vi "Init Edge Detector.vi"(6 "Unsee last word":bool=TRUE, 8 "error in (no error)":errorcluster, 11 "Spectrum Recorder too in":refnum<class "Spectrum Recorder too.lvclass">) -> (0 "error out":errorcluster, 3 "Spectrum Recorder too out":refnum<class "Spectrum Recorder too.lvclass">)   [LabVIEW 2018, in "Spectrum Recorder too.lvclass"]
uses:
  Spectrum Recorder too.lvclass
  Spectrum Recorder too.lvclass/Spectrum Recorder too.ctl
  Read RP transceiver.vi
  Write RP transceiver.vi
  NHMFL_Core/Libraries/Red Pitaya/RP Core/RP Transceiver/RP Transceiver.lvclass
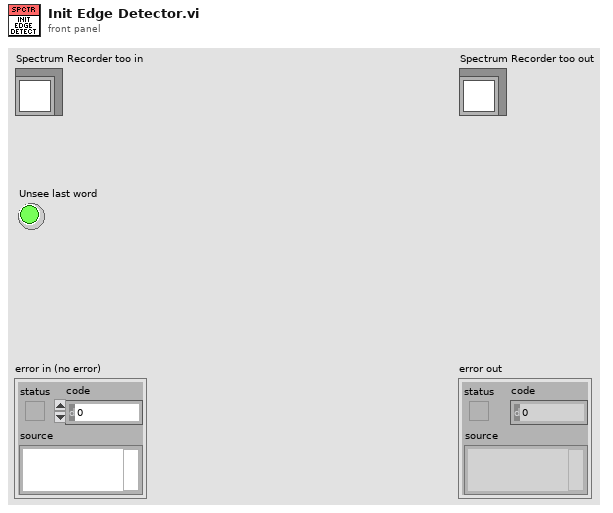
[diagram p1: front panel]
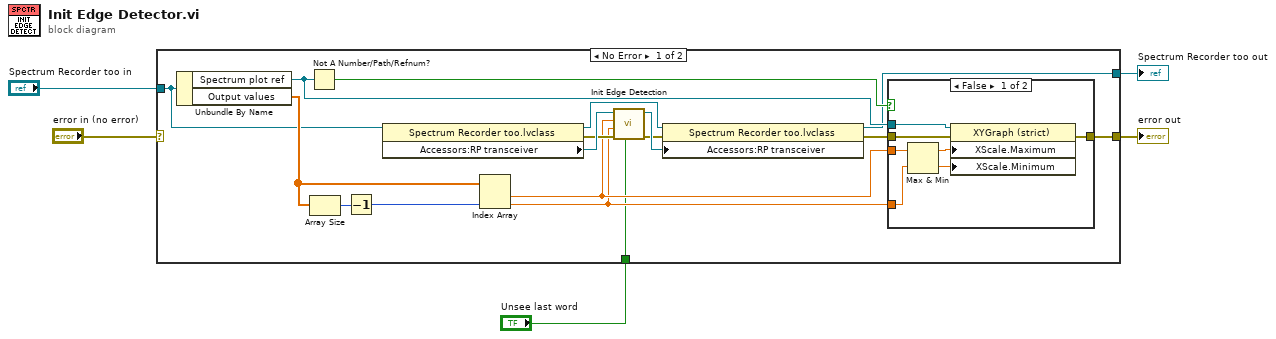
[diagram p0: block diagram]
diagram:
  n1 = case shown="No Error" "error in (no error)" {
    selector: "error in (no error)" -> [_ w32]
    tunnel: [w7 w32] -> w4
    tunnel: [w12 w31] -> w2
    tunnel: "Spectrum Recorder too in" -> [w13 w31]
    tunnel: "Unsee last word" -> [w6 _]
    frame No Error {
      n2 = Unbundle By Name(w13) -> ("Spectrum plot ref"=w18:refnum<vi>, "Output values"=w20:dbl[])
      n3 = Not A Number/Path/Refnum?(number/path/refnum=w18) -> (NaN/Path/Refnum?=w19:bool)
      n4 = Array Size(array=w20) -> (size(s)=w21:i32)
      n5 = Decrement(x=w21) -> (x-1=w22:i32)
      n6 = property class="Spectrum Recorder too.lvclass"(reference=w13) -> (reference out=w10:refnum<class "Spectrum Recorder too.lvclass">, error out=w15:errorcluster, "Accessors:RP transceiver"=w17:refnum<class "RP Transceiver.lvclass">)  [unwired: 1 in]
      n7 = Index Array(array=w20, index #2=w22) -> (element #1=w9:dbl, element #2=w8:dbl)  [unwired: 1 in]
      n8 = call-dynamic "Init Edge Detection.vi"("Unsee last word"=w6, "error in (no error)"=w15, "Last output"=w8, "First output"=w9, "RP Transceiver in"=w17) -> ("error out"=w11:errorcluster, "RP Transceiver out"=w16:refnum<class "RP Transceiver.lvclass">)  [unwired: 5 in]
      n9 = property class="Spectrum Recorder too.lvclass"(reference=w10, error in=w11, "Accessors:RP transceiver"=w16) -> (reference out=w12:refnum<class "Spectrum Recorder too.lvclass">, error out=w14:errorcluster)
      n10 = case shown="False" w19 {
        tunnel: w18 -> [w29 _]
        tunnel: w14 -> [w28 w30]
        tunnel: w9 -> [w27 _]
        tunnel: w8 -> [w26 _]
        tunnel: [w23 w30] -> w7
        frame False {
          n11 = Max & Min(x=w27, y=w26) -> (max(x,y)=w25:dbl, min(x,y)=w24:dbl)
          n12 = property class="XYGraph (strict)"(reference=w29, error in=w28, "XScale.Maximum"=w25, "XScale.Minimum"=w24) -> (error out=w23:errorcluster)  [unwired: 1 out]
        }
        frame True {
        }
      }
    }
    frame Error {
    }
  }
  "error out" <- w4
  "Spectrum Recorder too out" <- w2
